vi "module-04-or-nor.vi"() -> ()   [LabVIEW 2019]
panel:
  in  "Tab Control":enum32{"Execution", "Logic"}(tab)
  out "Digital State Chart":T1(graph)
  out "Ouptut":bool
  in  "Not Input 8":bool=TRUE
  in  "Not Input 7":bool=TRUE
  in  "Not Input 6":bool=TRUE
  in  "Not Input 5":bool=TRUE
  in  "Input 4":bool
  in  "Input 3":bool
  in  "Input 2":bool
  in  "Input":bool
  in  "Cycle \nMilliseconds":u32=100 min=10 max=30000 step=10
  # "OR NOR GATE TEST\nInputs 1-4 OR\nInputs 5-8 NOT  OR"
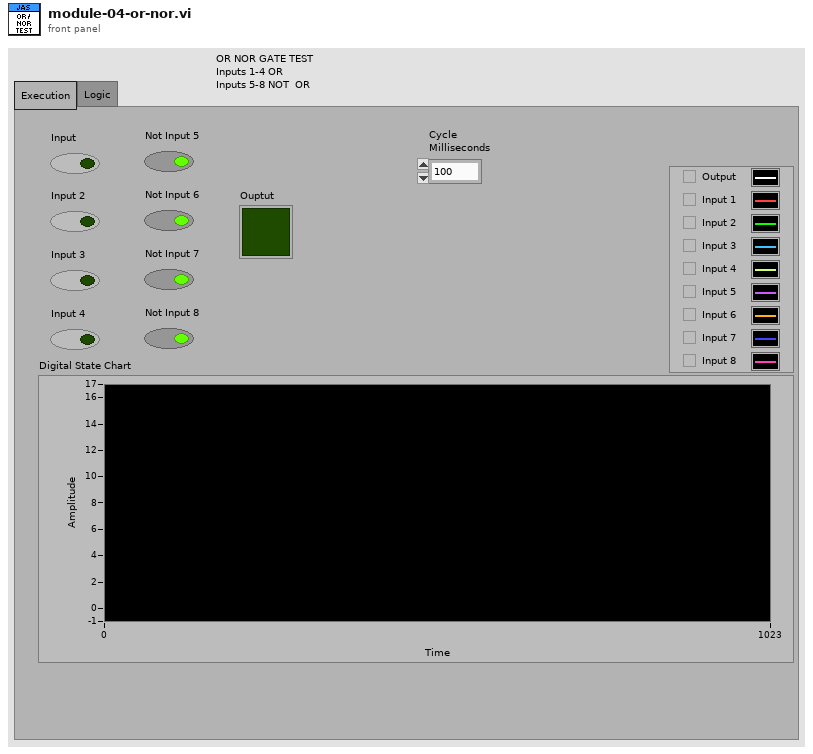
[diagram p1: front panel]
types:
  T1 = cluster{dbl, dbl, dbl, dbl, dbl, dbl, dbl, dbl, dbl}
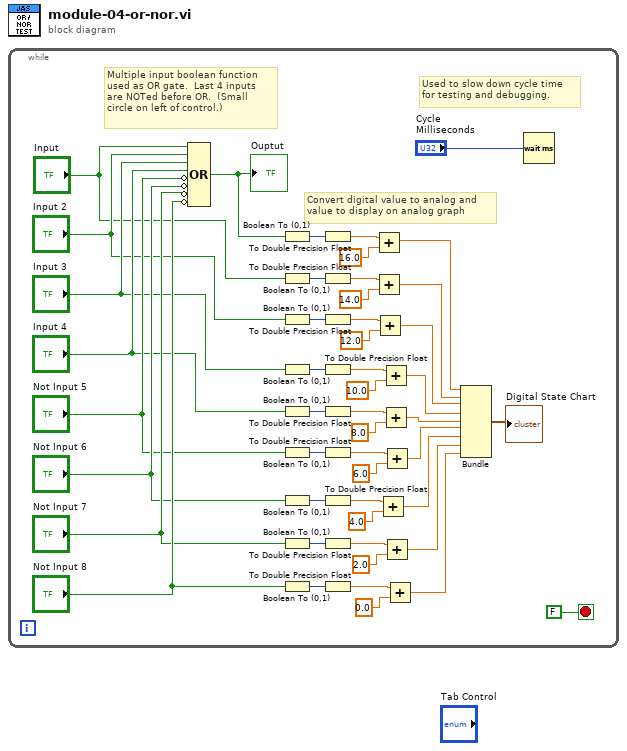
[diagram p0: block diagram]
diagram:
  n1 = while {
    stop <- FALSE stop-if-true
    # "Multiple input boolean function\nused as OR gate.  Last 4 inputs\nare NOTed before OR.  (Small\ncircle on left of control.)"
    # "Convert digital value to analog and \nvalue to display on analog graph"
    # "Used to slow down cycle time\nfor testing and debugging."
    n2 = Compound Arithmetic op=OR("Input", "Input 2", "Input 3", "Input 4", invert "Not Input 5", invert "Not Input 6", invert "Not Input 7", invert "Not Input 8") -> (w9:bool)
    "Ouptut" <- w9
    n3 = Boolean To (0,1)(Boolean=w9) -> (0, 1=w23:i16)
    n4 = Boolean To (0,1)(Boolean="Input") -> (0, 1=w24:i16)
    n5 = Boolean To (0,1)(Boolean="Input 2") -> (0, 1=w26:i16)
    n6 = Boolean To (0,1)(Boolean="Input 3") -> (0, 1=w35:i16)
    n7 = Boolean To (0,1)(Boolean="Input 4") -> (0, 1=w38:i16)
    n8 = Boolean To (0,1)(Boolean="Not Input 5") -> (0, 1=w40:i16)
    n9 = Boolean To (0,1)(Boolean="Not Input 6") -> (0, 1=w36:i16)
    n10 = Boolean To (0,1)(Boolean="Not Input 7") -> (0, 1=w42:i16)
    n11 = Boolean To (0,1)(Boolean="Not Input 8") -> (0, 1=w44:i16)
    n12 = To Double Precision Float(number=w23) -> (double precision float=w28:dbl)
    n13 = To Double Precision Float(number=w24) -> (double precision float=w25:dbl)
    n14 = To Double Precision Float(number=w26) -> (double precision float=w27:dbl)
    n15 = To Double Precision Float(number=w35) -> (double precision float=w46:dbl)
    n16 = To Double Precision Float(number=w38) -> (double precision float=w39:dbl)
    n17 = To Double Precision Float(number=w40) -> (double precision float=w41:dbl)
    n18 = To Double Precision Float(number=w36) -> (double precision float=w37:dbl)
    n19 = To Double Precision Float(number=w42) -> (double precision float=w43:dbl)
    n20 = To Double Precision Float(number=w44) -> (double precision float=w45:dbl)
    n21 = Add(x=w28, y=16.0) -> (x+y=w19:dbl)
    n22 = Add(x=w25, y=14.0) -> (x+y=w18:dbl)
    n23 = Add(x=w27, y=12.0) -> (x+y=w17:dbl)
    n24 = Add(x=w37, y=4.0) -> (x+y=w11:dbl)
    n25 = Add(x=w46, y=10.0) -> (x+y=w16:dbl)
    n26 = Add(x=w39, y=8.0) -> (x+y=w15:dbl)
    n27 = Add(x=w41, y=6.0) -> (x+y=w14:dbl)
    n28 = Add(x=w43, y=2.0) -> (x+y=w13:dbl)
    n29 = Add(x=w45, y=0.0) -> (x+y=w12:dbl)
    n30 = Bundle(w19, w18, w17, w16, w15, w14, w11, w13, w12) -> (→"Digital State Chart":T1)  [unwired: 1 in]
    n31 = Wait (ms)(milliseconds to wait="Cycle \nMilliseconds") -> ()  [unwired: 1 out]
  }
